vi "dataAcq_get_interferogram.vi"(0 "reference":refnum<class "OSA.lvclass">, 5 "error in (no error)":errorcluster) -> (14 "duplicate reference":refnum<class "OSA.lvclass">, 16 "saturated":bool, 19 "error out":errorcluster)   [LabVIEW 2010, in "OSA.lvclass"]
doc: "Reads data from spectrometer and updates labview buffer interferogram Y array, X is equidistant, (x min and max). See buffer_get.vi for labview buffer data access. \n\nX: optical path length\nY: ADC value"
uses:
  OSA.lvclass
  OSA20X_misc.lvlib
  FTSLib.dll
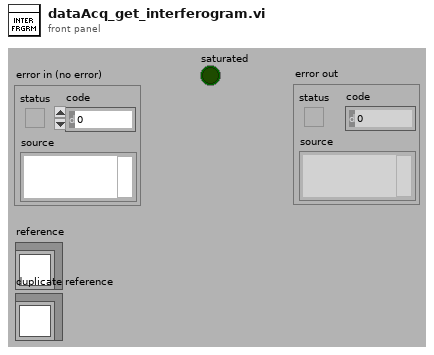
[diagram p1: front panel]
types:
  T1 = enum16{"get", "init", "set interferogram", "set spectrum", "cleanUp"}
  T2 = typedef "OSA.lvclass/ObjectAttributes.ctl" = cluster{"Stop":bool, "dataType":T3, "spectrometerIdx":u16, "buffer size interferogram":i32, "interferogram":cluster{"new":bool, "plot_x_ min":sgl, "plot_x_max":sgl, "plot_y_min":sgl, "plot_y_max":sgl, "Graph Intrfrgrm":T4, "timeStamp":u32, "signal (%)":dbl, "traces":cluster{"idx":u32, "broadBand":bool, "monoChromatic":bool, "peakToPeakSignal":dbl, "peakToPeakPos":dbl}[], "traces idx last":i32, "contrast (%)":dbl}, "spectrum":cluster{"new":bool, "plot_x_min":sgl, "plot_x_max":sgl, "plot_unit_x":T5, "plot_unit_y":T6, "plot_y_min":sgl, "plot_y_max":sgl, "Graph Spectrum":T4, "timeStamp":u32, "X_VAL_OPTIONS":enum16{"MIN_MAX", "ARRAY"}, "traces":cluster{"idx":u32}[], "traces idx last":i32}, "Thorlabs_OSA_64.lvclass:queue_action.ctlqueue ref":refnum<queue>, "action":T7, "plot zoom step":dbl, "buffer semaphore":T8, "acq stopped":bool, "dataType active":T3, "temperature (degr C)":sgl, "pressure (hPa)":sgl, "rel humidity (%)":sgl, "settings":cluster{"resolution":u16, "sensitivity":u16, "Average":bool, "average nr":u32, "apodisation":T9, "acq delay (ms)":u32, "airMesure":T10, "wmtr on":bool, "intfgrm_smooth_width":u16, "intfgrm_smooth_nrOfPasses":u16, "intfgrm_smooth":T11, "phaseCorrection":T12, "zeroFill":u8, "spectr_smooth":T11, "spectr_smooth_width":u16, "spectr_smooth_nrOfPasses":u16, "resolution (/cm)":sgl, "REF wavelength, (nm)":dbl, "gain_idx":u16, "gainAuto":bool, "gain_relative":dbl, "PD sensitivity mode":T13, "PD senseMode implemented":bool, "SensorTemperature implemented":bool, "SensorPressure implemented":bool, "SensorHumidity implemented":bool, "attenuationAuto":bool, "attenuationOnOff":bool, "attenuationAvailable":bool, "offsetAvailable":bool, "offset":i32, "offset max":u16, "contrastAvailable":bool}, "peaks position":sgl[], "peaks width":sgl[], "peaks height":sgl[], "peaks max nr":u32, "peaks latest nr":i32, "peaks new":bool, "power":dbl, "power new":bool, "path":string, "wavelength (WNr)":dbl, "wavelength new":bool, "buffer size spectrum":i32, "status":string, "vi reference":refnum<vi>, "funcPointer":u64, "libraryPointer":u64, "singleAcquisition":bool, "coherenceLength (cm)":dbl, "coherenceLength new":bool, "spectrometer model":string, "spectrometer serial nr":string, "peaks thld left":sgl[], "peaks thld right":sgl[], "coherenceLength error (cm)":dbl, "ADC bits":u16, "peaks position centroid":sgl[], "peaks height centroid":sgl[], "OSA series":T14, "channel index spectrum":u16, "spectrometer rangeLow, (/cm)":dbl, "spectrometer rangeHigh, (/cm)":dbl, "channel index interferogram":u16, "virtualSource":bool, "sweep restart":bool}
  T3 = typedef "OSA.lvclass/acq_dataType.ctl" = enum16{"none", "interferogram", "spectrum"}
  T4 = typedef "OSA.lvclass/graph_intensity.ctl" = refnum<vi>
  T5 = typedef "OSA.lvclass/spectrum_x_unit.ctl" = enum16{"wavenr/cm", "THz", "eV", "nm_air", "nm_vac"}
  T6 = typedef "OSA.lvclass/y_unit.ctl" = enum16{"ADC counts", "dBm pwr absolute", "dBm pwr density", "mW pwr absolute", "mW pwr density"}
  T7 = typedef "OSA.lvclass/queue_action.ctl" = enum16{"none", "stop", "GUI_plotInterferogram", "GUI_plotSpectrum", "GUI_plotInterferogramRescale", "GUI_plotSpectrumRescale", "GUI_plotInterferogramReset", "GUI_plotSpectrumReset", "GUI_plotInterferogramAutoScaleY", "GUI_plotSpectrumAutoScaleY", "GUI_plotInterferogramZoomOut", "GUI_plotSpectrumZoomOut", "GUI_plotInterferogramPane", "GUI_plotSpectrumPane", "GUI_plotInterferogramZoomMouse", "GUI_plotSpectrumZoomMouse", "GUI_plotSpectrumFSRY", "GUI_plotInterferogramFSRY", "GUI_spectrumChannelType", "GUI_channel", "ENVIRONMENT temperature", "ENVIRONMENT pressure", "MODE_resolution set", "MODE_resolution get", "MODE_sensitivity set", "MODE_sensitivity get", "MODE_PDTemperature set", "MODE_PDTemperature get", "REBOOT/RESET firmware", "ACQASYNC_acquireSingleSpectrum", "ACQASYNC_continuous start", "ACQASYNC_continuous stop\n", "ACQASYNC_get last interferogram", "ACQASYNC_get last spectrum", "ACQASYNC_get last waveNr", "ACQOPT_interferogram smoothing set", "ACQOPT_interferogram smoothing get", "ACQOPT_spectrum smoothing set", "ACQOPT_spectrum smoothing get", "ACQOPT_apodisation type set", "ACQOPT_apodisation type get", "ACQOPT_phase correction type set", "ACQOPT_phase correction type get", "ACQOPT_acqIntervall_set", "ACQOPT_acqIntervall_get", "ACQOPT_average spectrum set", "ACQOPT_average spectrum get", "ACQOPT_rolling average set", "ACQOPT_rolling average get", "ACQOPT_zero fill factor set", "ACQOPT_zero fill factor get", "ACQOPT_cycle counting set", "ACQOPT_cycle counting get", "ACQOPT_air measure option set", "ACQOPT_air measure option get", "ACQOPT_gainLevel auto get", "ACQOPT_gainLevel auto set", "ACQOPT_gainLevel get", "ACQOPT_gainLevel set", "ACQOPT_offset set", "ACQOPT_attenuator_auto_set", "ACQOPT_attenuator_set", "ACQOPT_getAll", "INSTRUMENT_PROPERTY_range_WaveNr_min", "INSTRUMENT_PROPERTY_range_WaveNr_max", "INSTRUMENT_PROPERTY_reference_wavelength_cm^-1", "INSTRUMENT_PROPERTY_samplesPerRefPeriod", "INSTRUMENT_PROPERTY_resolution_waveNrPercm", "INSTRUMENT_PROPERTY_availableGainLevels", "INSTRUMENT_PROPERTY_status", "CONVERT", "ANALYSE_POWER", "ANALYSE_PEAKS", "ANALYSE_WAVELENGTH", "ANALYSE_SPECTRUM", "ANALYSE_INTERFEROGRAM", "ANALYSE_COHERENCE_LENGTH", "MATH", "MATH_power", "MATH_peaks", "FILE", "miscellaneous"}
  T8 = typedef "Semaphore RefNum" = refnum<k1>
  T9 = typedef "OSA.lvclass/apodisation.ctl" = enum16{"NONE", "NORTON_BEER_WEAK", "NORTON_BEER_MEDIUM", "NORTON_BEER_STRONG", "TRIANGULAR", "COSINE", "HANN", "HAMMING", "BLACKMANHARRIS3", "BLACKMANHARRIS4", "GAUSSIAN"}
  T10 = typedef "OSA.lvclass/airMeasure.ctl" = enum16{"TEMPERATURE", "PRESSURE"}
  T11 = typedef "OSA20X_misc.lvlib/interferogram_smoothing.ctl" = enum16{"NONE", "BINOMIAL", "SAVITSKY_GOLAY", "FOURIER", "MOVING_AVERAGE", "GAUSSIAN"}
  T12 = typedef "OSA.lvclass/phaseCorrection.ctl" = enum16{"NONE", "MERTZ", "FORMAN", "MERTZ_FILE", "FORMAN_FILE", "FUTURE COMP."}
  T13 = typedef "OSA20X_misc.lvlib/PDTemperatureMode.ctl" = enum16{"cool: better sensitivity/noise floor", "warm: extended wl range"}
  T14 = typedef "OSA.lvclass/OSA_series.ctl" = enum16{"OSA200", "OSA300", "UNKNOWN"}
  T15 = typedef "OSA.lvclass/interferogram_properties.ctl" = cluster{"length":u32, "X min (cm)":sgl, "X max (cm)":sgl, "saturated":bool, "broadband":bool, "isMonoChromatic":bool, "peakToPeak, (counts)":dbl, "peakToPeak position (cm)":dbl, "samplesPerRefPeriod":sgl, "OPDmin (cm)":sgl, "OPDmax (cm)":sgl, "contrast":dbl}
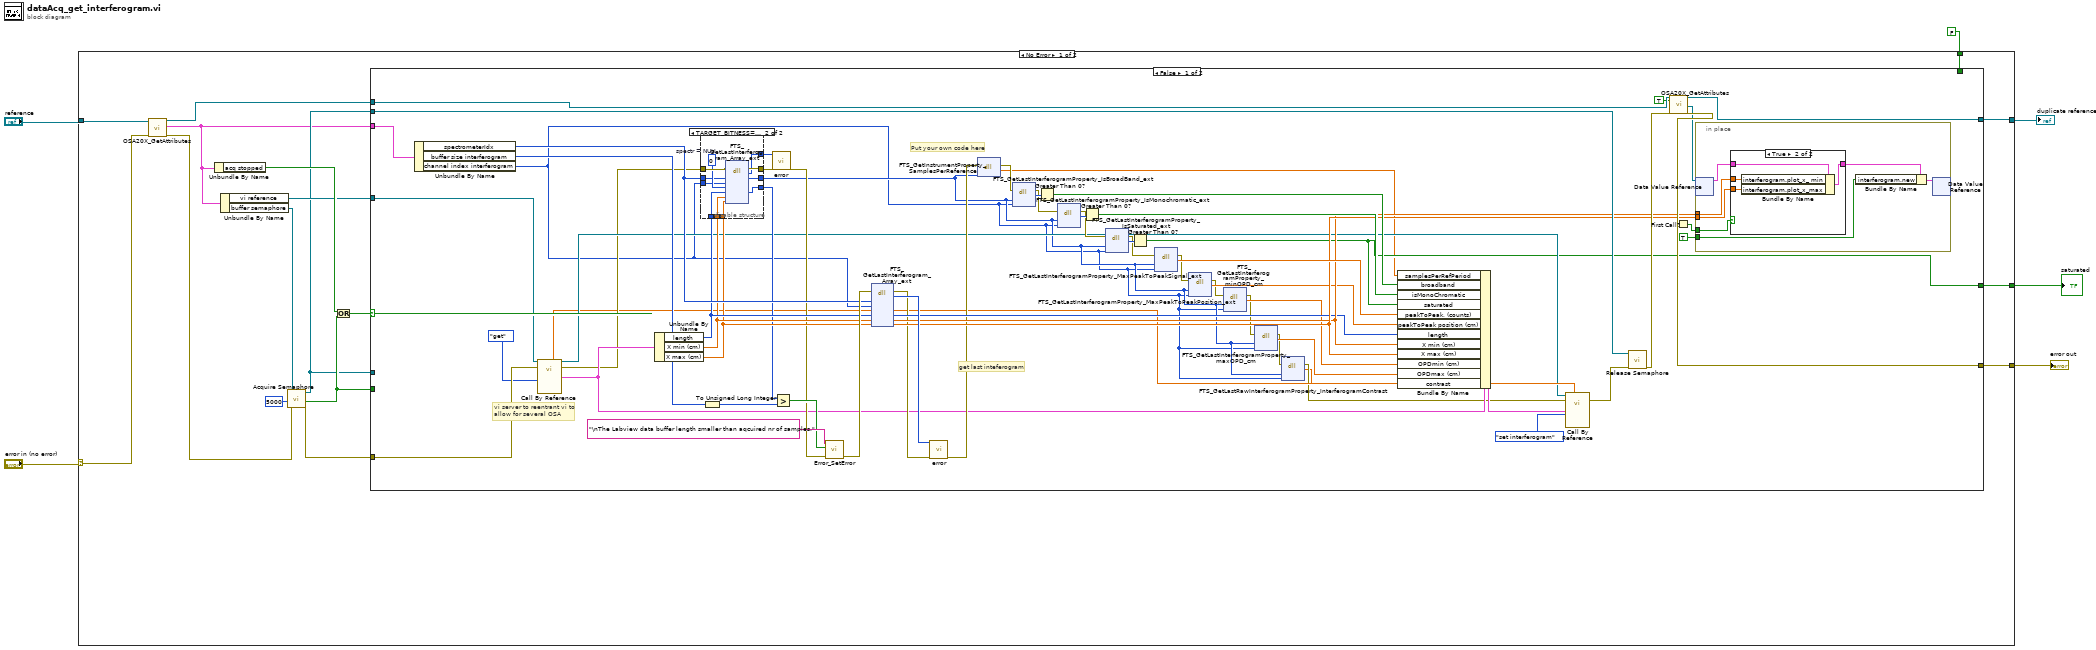
[diagram p0: block diagram]
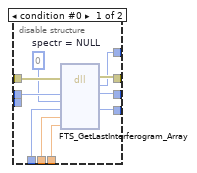
[diagram p2: hidden frame]
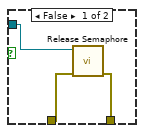
[diagram p5: hidden frame]
diagram:
  n1 = case shown="No Error" "error in (no error)" {
    selector: "error in (no error)" -> [w22 w132]
    tunnel: [w21 w132] -> w5
    tunnel: "reference" -> [w23 w131]
    tunnel: [w20 w131] -> w3
    tunnel: [w8 w130] -> w2
    tunnel: FALSE -> [w7 w130]
    frame No Error {
      n2 = call "OSA20X_GetAttributes.vi"("reference in"=w23, "error in (no error)"=w22) -> ("reference out"=w12:refnum<class "OSA.lvclass">, "Data"=w9:T2, "error out"=w16:errorcluster)  [unwired: 14 in, 1 out]
      n3 = Unbundle By Name(w9) -> ("acq stopped"=w19:bool)
      n4 = Unbundle By Name(w9) -> ("vi reference"=w13:refnum<vi>, "buffer semaphore"=w17:T8)
      n5 = call <vilib>:"Acquire Semaphore.vi"("error in (no error)"=w16, "ms timeout (-1)"=5000, "semaphore"=w17) -> ("error out"=w14:errorcluster, "timed out"=w11:bool, "semaphore out"=w10:T8)  [unwired: 2 in]
      n6 = Or(x=w19, y=w11) -> (x .or. y?=w18:bool)
      n7 = case shown="False" w18 {
        tunnel: w9 -> [w86 _]
        tunnel: w14 -> [w33 w122]
        tunnel: [w83 w121] -> w21
        tunnel: [w82 w125] -> w20
        tunnel: w10 -> [w77 _]
        tunnel: w13 -> [w37 _]
        tunnel: w12 -> [w76 w125]
        tunnel: w11 -> [_ w124]
        tunnel: w10 -> [_ w123]
        tunnel: [w25 w120] -> w8
        tunnel: w7 -> [_ w120]
        frame False {
          # "get last inteferogram"
          # "vi server to reentrant vi to \nallow for several OSA"
          # "Put your own code here"
          n8 = Unbundle By Name(w86) -> ("spectrometerIdx"=w53:u16, "buffer size interferogram"=w80:i32, "channel index interferogram"=w26:u16)
          n9 = call-by-ref "?"(reference=w37, error in=w33, "action"=T1."get") -> (reference out=w36:refnum<vi>, error out=w34:errorcluster, "interferogram"=w31:sgl[], "interferogram prop"=w35:T15)  [unwired: 14 in, 3 out]
          n10 = Unbundle By Name(w35) -> ("length"=w52:u32, "X min (cm)"=w51:sgl, "X max (cm)"=w50:sgl)
          n11 = disable-structure shown="TARGET_BITNESS==64, default" {
            disable-tunnel: w34 -> [w95 w107]
            disable-tunnel: [w94 w106] -> w48
            disable-tunnel: w53 -> [w96 w104]
            disable-tunnel: [w89 w103] -> w30
            disable-tunnel: w52 -> [w91 w102]
            disable-tunnel: w51 -> [w92 w101]
            disable-tunnel: w50 -> [w93 w100]
            disable-tunnel: [w90 w99] -> w49
            disable-tunnel: [w87 w98] -> w46
            disable-tunnel: w26 -> [_ w97]
            frame condition #0 {
              w88 = u32 0  # spectr = NULL
              n12 = dll-call lib="FTSLib.dll" fn="FTS_GetLastInterferogram_Array"(error in=w95, "spectrIdx"=w96, "spec"=w88, "length"=w91, "x_min"=w92, "x_max"=w93) -> (error out=w94:errorcluster, "return type"=w87:i32, "spectrIdx"=w89:u16, "length"=w90:u32)  [unwired: 5 in, 1 out]
            }
            frame condition #1 (active) {
              w105 = u64 0  # spectr = NULL
              n13 = dll-call lib="FTSLib.dll" fn="FTS_GetLastInterferogram_Array_ext"(error in=w107, "spectrIdx"=w104, "channel"=w97, "spec"=w105, "length"=w102, "x_min"=w101, "x_max"=w100) -> (error out=w106:errorcluster, "return type"=w98:i32, "spectrIdx"=w103:u16, "length"=w99:u32)  [unwired: 6 in, 1 out]
            }
          }
          n14 = To Unsigned Long Integer(number=w80) -> (unsigned 32bit integer=w79:u32)
          n15 = call "error.vi"("result code"=w46, "error in (no error)"=w48) -> ("error out"=w47:errorcluster)  [unwired: 15 in, 2 out]
          n16 = Greater?(x=w49, y=w79) -> (0:w84:bool)
          n17 = call "Error_SetError.vi"("error in"=w47, "status (true)"=w84, "source(\"\")"="\nThe Labview data buffer length smaller than aqcuired nr of samples." ("source(\"\")")) -> ("error out"=w55:errorcluster)  [unwired: 4 in]
          n18 = dll-call lib="FTSLib.dll" fn="FTS_GetLastInterferogram_Array_ext"(error in=w55, "spectrIdx"=w53, "channel"=w26, "spec"=w31, "length"=w52, "x_min"=w51, "x_max"=w50) -> (error out=w56:errorcluster, "return type"=w81:i32, "spec"=w38:sgl[], "length"=w59:u32, "x_min"=w60:sgl, "x_max"=w61:sgl)  [unwired: 4 in, 1 out]
          n19 = call "error.vi"("result code"=w81, "error in (no error)"=w56) -> ("error out"=w54:errorcluster)  [unwired: 15 in, 2 out]
          n20 = dll-call lib="FTSLib.dll" fn="FTS_GetInstrumentProperty_SamplesPerReference"(error in=w54, "spectrIdx"=w30) -> (error out=w57:errorcluster, "return type"=w24:sgl)  [unwired: 3 in, 1 out]
          n21 = dll-call lib="FTSLib.dll" fn="FTS_GetLastInterferogramProperty_IsBroadBand_ext"(error in=w57, "spectrIdx"=w30, "channel"=w26) -> (error out=w69:errorcluster, "return type"=w71:u8)  [unwired: 4 in, 1 out]
          n22 = Greater Than 0?(x=w71) -> (x > 0?=w70:bool)
          n23 = dll-call lib="FTSLib.dll" fn="FTS_GetLastInterferogramProperty_IsMonochromatic_ext"(error in=w69, "spectrIdx"=w30, "channel"=w26) -> (error out=w66:errorcluster, "return type"=w68:u8)  [unwired: 4 in, 1 out]
          n24 = Greater Than 0?(x=w68) -> (x > 0?=w67:bool)
          n25 = dll-call lib="FTSLib.dll" fn="FTS_GetLastInterferogramProperty_IsSaturated_ext"(error in=w66, "spectrIdx"=w30, "channel"=w26) -> (error out=w64:errorcluster, "return type"=w65:u8)  [unwired: 4 in, 1 out]
          n26 = Greater Than 0?(x=w65) -> (x > 0?=w25:bool)
          n27 = dll-call lib="FTSLib.dll" fn="FTS_GetLastInterferogramProperty_MaxPeakToPeakSignal_ext"(error in=w64, "spectrIdx"=w30, "channel"=w26) -> (error out=w62:errorcluster, "return type"=w63:dbl)  [unwired: 4 in, 1 out]
          n28 = dll-call lib="FTSLib.dll" fn="FTS_GetLastInterferogramProperty_MaxPeakToPeakPosition_ext"(error in=w62, "spectrIdx"=w30, "channel"=w26) -> (error out=w45:errorcluster, "return type"=w58:dbl)  [unwired: 4 in, 1 out]
          n29 = dll-call lib="FTSLib.dll" fn="FTS_GetLastInterferogramProperty_minOPD_cm"(error in=w45, "spectrIdx"=w30, "channel"=w26) -> (error out=w43:errorcluster, "return type"=w44:dbl)  [unwired: 4 in, 1 out]
          n30 = dll-call lib="FTSLib.dll" fn="FTS_GetLastInterferogramProperty_maxOPD_cm"(error in=w43, "spectrIdx"=w30, "channel"=w26) -> (error out=w29:errorcluster, "return type"=w42:dbl)  [unwired: 4 in, 1 out]
          n31 = dll-call lib="FTSLib.dll" fn="FTS_GetLastRawInterferogramProperty_InterferogramContrast"(error in=w29, "spectrIdx"=w30, "channel"=w26) -> (error out=w28:errorcluster, "return type"=w27:dbl)  [unwired: 4 in, 1 out]
          n32 = Bundle By Name(cluster=w35, "samplesPerRefPeriod"=w24, "broadband"=w70, "isMonoChromatic"=w67, "saturated"=w25, "peakToPeak, (counts)"=w63, "peakToPeak position (cm)"=w58, "length"=w59, "X min (cm)"=w60, "X max (cm)"=w61, "OPDmin (cm)"=w44, "OPDmax (cm)"=w42, "contrast"=w27) -> (w40:T15)
          n33 = call-by-ref "?"(reference=w36, error in=w28, "interferogram prop set"=w40, "action"=T1."set interferogram", "interferogram set"=w38) -> (error out=w41:errorcluster)  [unwired: 12 in, 6 out]
          n34 = call <vilib>:"Release Semaphore.vi"("error in (no error)"=w41, "semaphore"=w77) -> ("error out"=w78:errorcluster)  [unwired: 4 in, 1 out]
          n35 = call "OSA20X_GetAttributes.vi"("reference in"=w76, "OnlyGetDvrReference(False)"=TRUE, "error in (no error)"=w78) -> ("reference out"=w82:refnum<class "OSA.lvclass">, "DataRef"=w74:refnum<data-value>, "error out"=w83:errorcluster)  [unwired: 13 in, 1 out]
          n36 = First Call?() -> (First Call?: T/F=w73:bool)
          n37 = in-place {
            in-place-border: w73 -> [w114]
            in-place-border: w60 -> [w112]
            in-place-border: w61 -> [w111]
            in-place-border: TRUE ("interferogram.new") -> [w109]
            n38 = in-place-dvr #1(w74) -> (w113:T2)  [unwired: 1 out]
            n39 = case shown="True" w114 {
              tunnel: w113 -> [w115 w119]
              tunnel: [w115 w118] -> w110
              tunnel: w112 -> [_ w117]
              tunnel: w111 -> [_ w116]
              frame False {
              }
              frame True {
                n40 = Bundle By Name(cluster=w119, "interferogram.plot_x_ min"=w117, "interferogram.plot_x_max"=w116) -> (w118:T2)
              }
            }
            n41 = Bundle By Name(cluster=w110, "interferogram.new"=w109) -> (w108:T2)
            n42 = in-place-dvr #1(w108) -> ()  [unwired: 2 out]
          }
        }
        frame True {
          n43 = case shown="True" w124 {
            tunnel: w123 -> [w128 _]
            tunnel: w122 -> [w127 w129]
            tunnel: [w126 w129] -> w121
            frame False {
              n44 = call <vilib>:"Release Semaphore.vi"("error in (no error)"=w127, "semaphore"=w128) -> ("error out"=w126:errorcluster)  [unwired: 4 in, 1 out]
            }
            frame True {
            }
          }
        }
      }
    }
    frame Error {
      # "Error"
    }
  }
  "error out" <- w5
  "duplicate reference" <- w3
  "saturated" <- w2
